vi "test teleop.vi"(11 "Boolean":bool) -> (3 "Numeric":dbl)   [LabVIEW 2019]
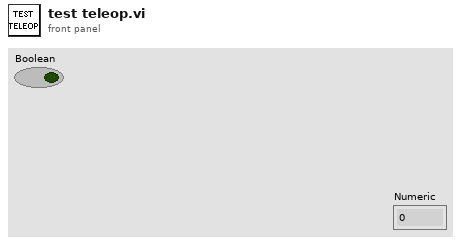
[diagram p1: front panel]
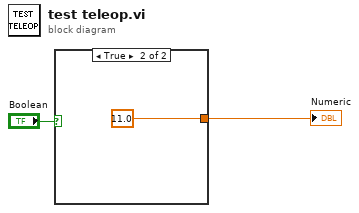
[diagram p0: block diagram]
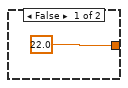
[diagram p2: hidden frame]
diagram:
  n1 = case shown="True" "Boolean" {
    tunnel: [22.0 ("Numeric") 11.0 ("Numeric")] -> w2
    frame False {
    }
    frame True {
    }
  }
  "Numeric" <- w2
